vi "Set Switch Pin High.vi"(8 "error in (no error)":errorcluster, 10 "Pin":u16, 11 "PEU in":refnum<class "PEU.lvclass">) -> (0 "error out":errorcluster, 3 "PEU out":refnum<class "PEU.lvclass">)   [LabVIEW 2020, in "PEU.lvlib" / "PEU.lvclass"]
uses:
  PEU.lvclass
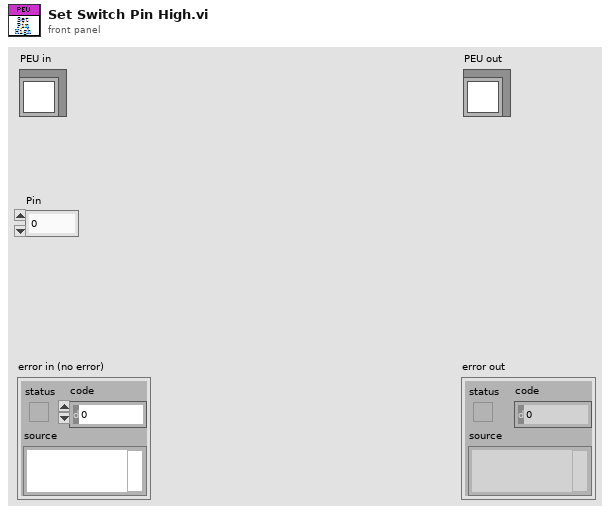
[diagram p1: front panel]
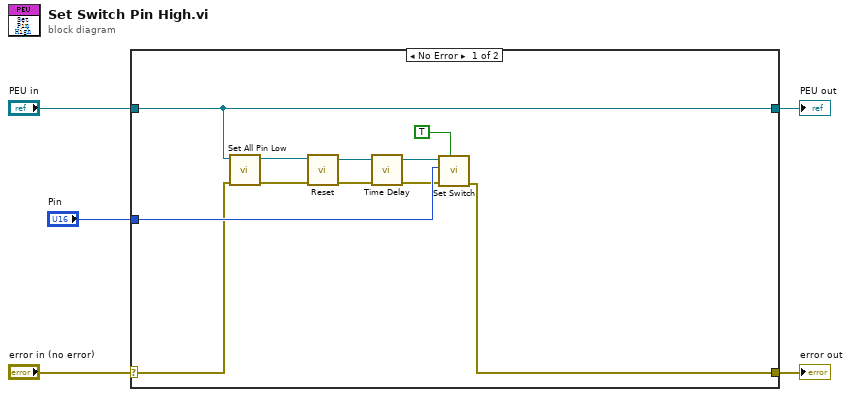
[diagram p0: block diagram]
diagram:
  n1 = case shown="No Error" "error in (no error)" {
    selector: "error in (no error)" -> [w9 w17]
    tunnel: [w8 w17] -> w4
    tunnel: [w15 w16] -> w2
    tunnel: "PEU in" -> [w15 w16]
    tunnel: "Pin" -> [w10 _]
    frame No Error {
      n2 = call "Set All Pin Low.vi"("error in (no error)"=w9, "PEU in"=w15) -> ("error out"=w13:errorcluster, "PEU out"=w14:refnum<class "PEU.lvclass">)  [unwired: 8 in]
      n3 = call "Reset.vi"("error in (no error)"=w13, "PEU in"=w14) -> ("error out"=w7:errorcluster, "PEU out"=w12:refnum<class "PEU.lvclass">)  [unwired: 8 in]
      n4 = call "Time Delay"("error in (no error)"=w7) -> ("error out"=w6:errorcluster)  [unwired: 10 in]
      n5 = call "Set Switch.vi"("ON/OFF"=TRUE, "error in (no error)"=w6, "Pin"=w10, "PEU in"=w12) -> ("error out"=w8:errorcluster)  [unwired: 6 in, 1 out]
    }
    frame Error {
    }
  }
  "error out" <- w4
  "PEU out" <- w2
